vi "Read Duration.vi"(8 "error in (no error)":errorcluster, 11 "Write Duration Msg in":refnum<class "Write Duration Msg.lvclass">) -> (0 "error out":errorcluster, 2 "Duration":dbl, 3 "Write Duration Msg out":refnum<class "Write Duration Msg.lvclass">)   [LabVIEW 2015, in "Write Duration Msg.lvclass"]
uses:
  Write Duration Msg.lvclass
  Write Duration Msg.lvclass/Write Duration Msg.ctl
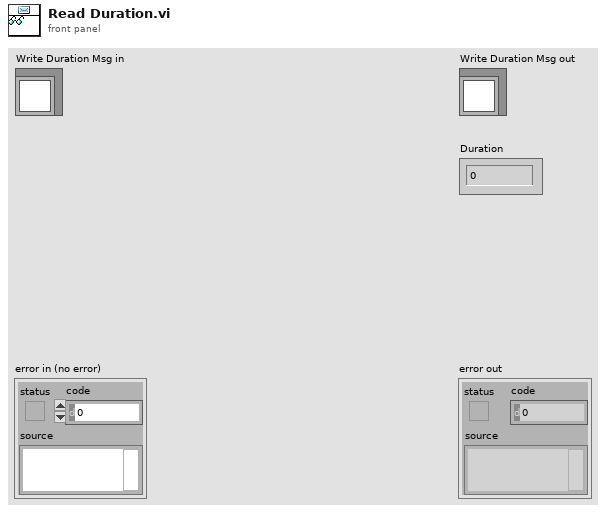
[diagram p1: front panel]
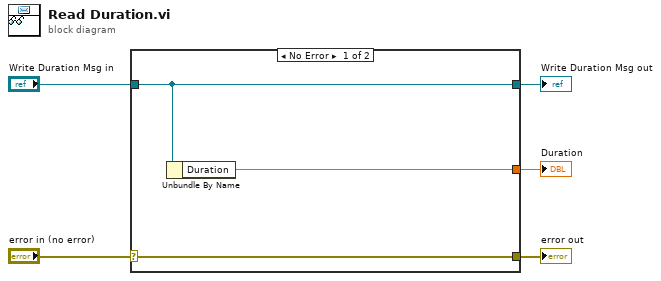
[diagram p0: block diagram]
diagram:
  n1 = case shown="No Error" "error in (no error)" {
    selector: "error in (no error)" -> [w8 w9]
    tunnel: [w8 w9] -> w4
    tunnel: [w7 w10] -> w2
    tunnel: "Write Duration Msg in" -> [w7 w10]
    tunnel: [w6 _] -> w1
    frame No Error {
      n2 = Unbundle By Name(w7) -> ("Duration"=w6:dbl)
    }
    frame Error {
    }
  }
  "error out" <- w4
  "Write Duration Msg out" <- w2
  "Duration" <- w1
